vi "Send Shutdown Command.vi"(8 "error in (no error)":errorcluster, 11 "Transceiver Interface in":refnum<class "Transceiver Interface.lvclass">) -> (0 "error out":errorcluster, 3 "Transceiver Interface out":refnum<class "Transceiver Interface.lvclass">)   [LabVIEW 2017, in "Data Sharing Framework Core.lvlib" / "Data Sharing Framework Engine.lvlib" / "Transceiver Thread.lvclass"]
uses:
  Transceiver Thread.lvclass
  Interfaces/Transceiver Interface/Transceiver Interface.lvclass
  Interfaces/Transceiver Interface/Command Data.ctl
  Interfaces/Transceiver Interface/Command.ctl
  Interfaces/Transceiver Interface/Command Parameters.ctl
  Interfaces/Transceiver Interface/Response.ctl
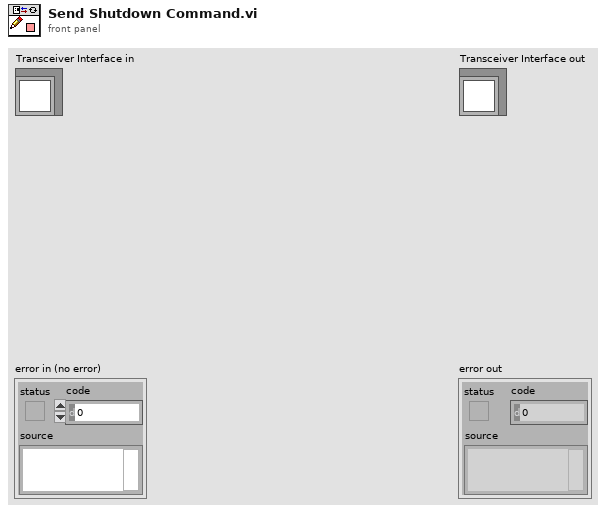
[diagram p1: front panel]
types:
  T1 = typedef "Data Sharing Framework Core.lvlib/Data Sharing Framework Engine.lvlib/Transceiver Interface.lvclass/Command Data.ctl" = cluster{"Command":T2, "Command Parameters":T3}
  T2 = typedef "Data Sharing Framework Core.lvlib/Data Sharing Framework Engine.lvlib/Transceiver Interface.lvclass/Command.ctl" = enum8{"Set Base Pointer", "Receive", "Transmit", "Shutdown"}
  T3 = typedef "Data Sharing Framework Core.lvlib/Data Sharing Framework Engine.lvlib/Transceiver Interface.lvclass/Command Parameters.ctl" = cluster{"arg1":u64, "arg2":u64}
  T4 = typedef "Data Sharing Framework Core.lvlib/Data Sharing Framework Engine.lvlib/Transceiver Interface.lvclass/Response.ctl" = enum8{"General Ack", "Shutting Down"}
  T5 = typedef "Data Sharing Framework Core.lvlib/Data Sharing Framework Engine.lvlib/Transceiver Interface.lvclass/Response Data.ctl" = cluster{"Response":T4, "Response Parameters":T6}
  T6 = typedef "Data Sharing Framework Core.lvlib/Data Sharing Framework Engine.lvlib/Transceiver Interface.lvclass/Response Parameters.ctl" = cluster{"arg1":u64, "arg2":u64}
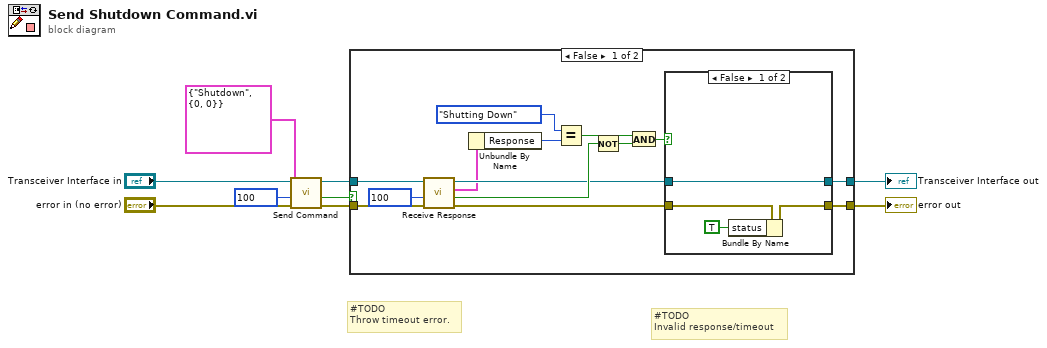
[diagram p0: block diagram]
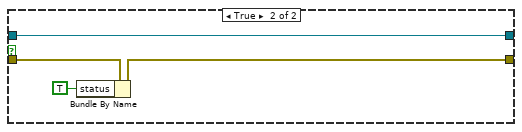
[diagram p3: hidden frame]
diagram:
  # "#TODO\nInvalid response/timeout"
  # "#TODO\nThrow timeout error."
  n1 = call "Send Command.vi"("error in (no error)"="error in (no error)", "timeout in ms (0)"=100, "command"=T1 {"Command"=enum."Shutdown", "Command Parameters"={"arg1"=0, "arg2"=0}}, "Transceiver Interface in"="Transceiver Interface in") -> ("error out"=w6:errorcluster, "timed out?"=w7:bool, "Transceiver Interface out"=w5:refnum<class "Transceiver Interface.lvclass">)  [unwired: 5 in]
  n2 = case shown="False" w7 {
    tunnel: w6 -> [w22 w33]
    tunnel: w5 -> [w23 w30]
    tunnel: [w13 w31] -> w2
    tunnel: [w11 w30] -> w1
    frame False {
      n3 = call "Receive Response.vi"("error in (no error)"=w22, "timeout in ms (0)"=100, "Transceiver Thread in"=w23) -> ("error out"=w14:errorcluster, "timed out?"=w18:bool, "response"=w10:T5, "Transceiver Thread out"=w12:refnum<class "Transceiver Interface.lvclass">)  [unwired: 5 in]
      n4 = Unbundle By Name(w10) -> ("Response"=w20:T4)
      n5 = Equal?(x=Response."Shutting Down", y=w20) -> (x = y?=w17:bool)
      n6 = Not(x=w18) -> (.not. x?=w16:bool)
      n7 = And(x=w17, y=w16) -> (x .and. y?=w15:bool)
      n8 = case shown="False" w15 {
        tunnel: w14 -> [w27 w29]
        tunnel: [w25 w29] -> w13
        tunnel: w12 -> [w24 w28]
        tunnel: [w24 w28] -> w11
        frame False {
          n9 = Bundle By Name(cluster=w27, "status"=TRUE) -> (w25:errorcluster)
        }
        frame True {
        }
      }
    }
    frame True {
      n10 = Bundle By Name(cluster=w33, "status"=TRUE) -> (w31:errorcluster)
    }
  }
  "error out" <- w2
  "Transceiver Interface out" <- w1
